vi "Depth and Stainless Correction Pop Up.vi"(2 "New Number\n of Stainless\n(Count)":i32, 3 "Input \nCorrected \nDepth (Feet)":sgl format="%.2f") -> (0 "Feet of\nStainless to be\nUsed (Count)":i32, 1 "Depth to \nbe Used \n(Feet)":sgl format="%.2f")   [LabVIEW 2016]
doc: "This vi allows the clinician to input the starting flexion. It used in order to derive a flexion correction."
panel:
  out "Original \nUncorrected \nDepth (Feet)":sgl format="%.2f"
  out "Original Feet\n of Stainless\n(Count)":i32
  in  "stop":bool
  in  "Increment Stainless":bool
  in  "Stainless OK As Is":bool
  in  "Correct Stainless":bool
  in  "Depth OK As Is":bool
  in  "Correct Depth":bool
  # "Please Choose \nto Correct Depth\nor to Leave As Is"
  # "Please Choose \nto Correct, Increment, or to \nLeave Feet of Stainless as is"
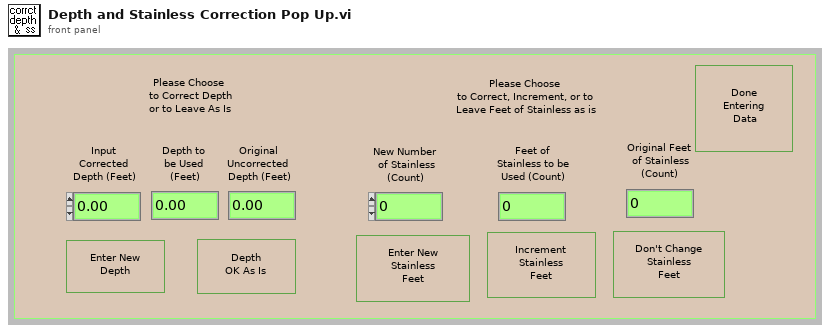
[diagram p1: front panel]
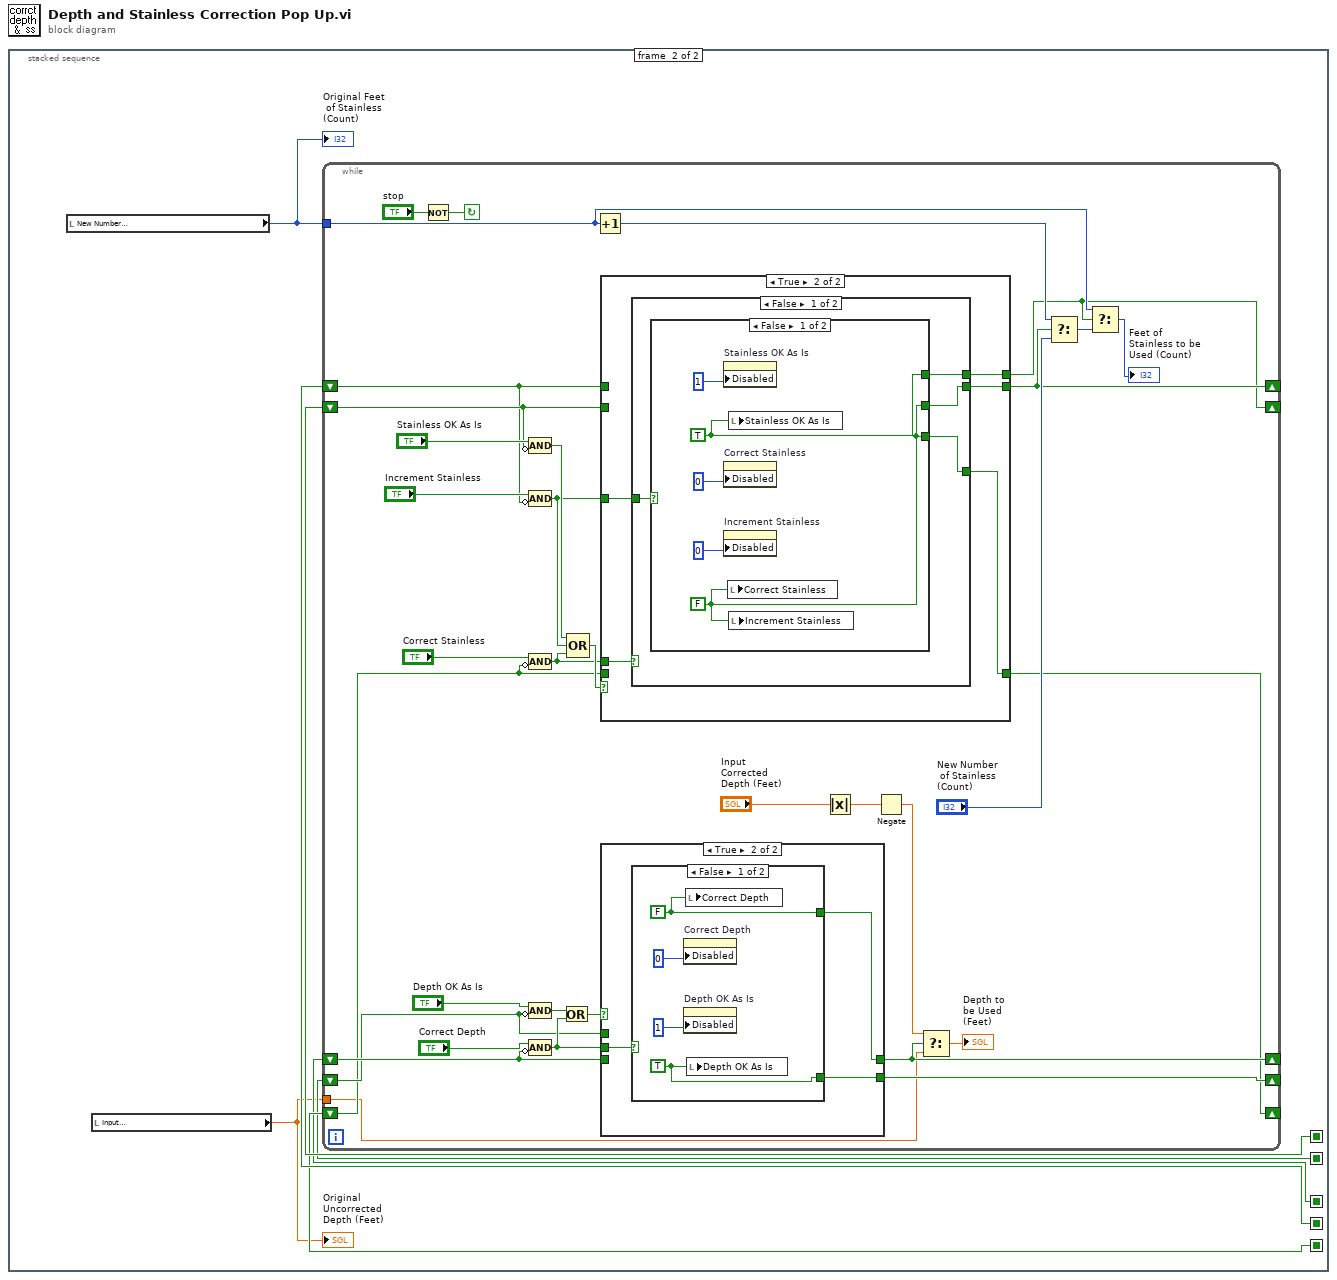
[diagram p0: block diagram]
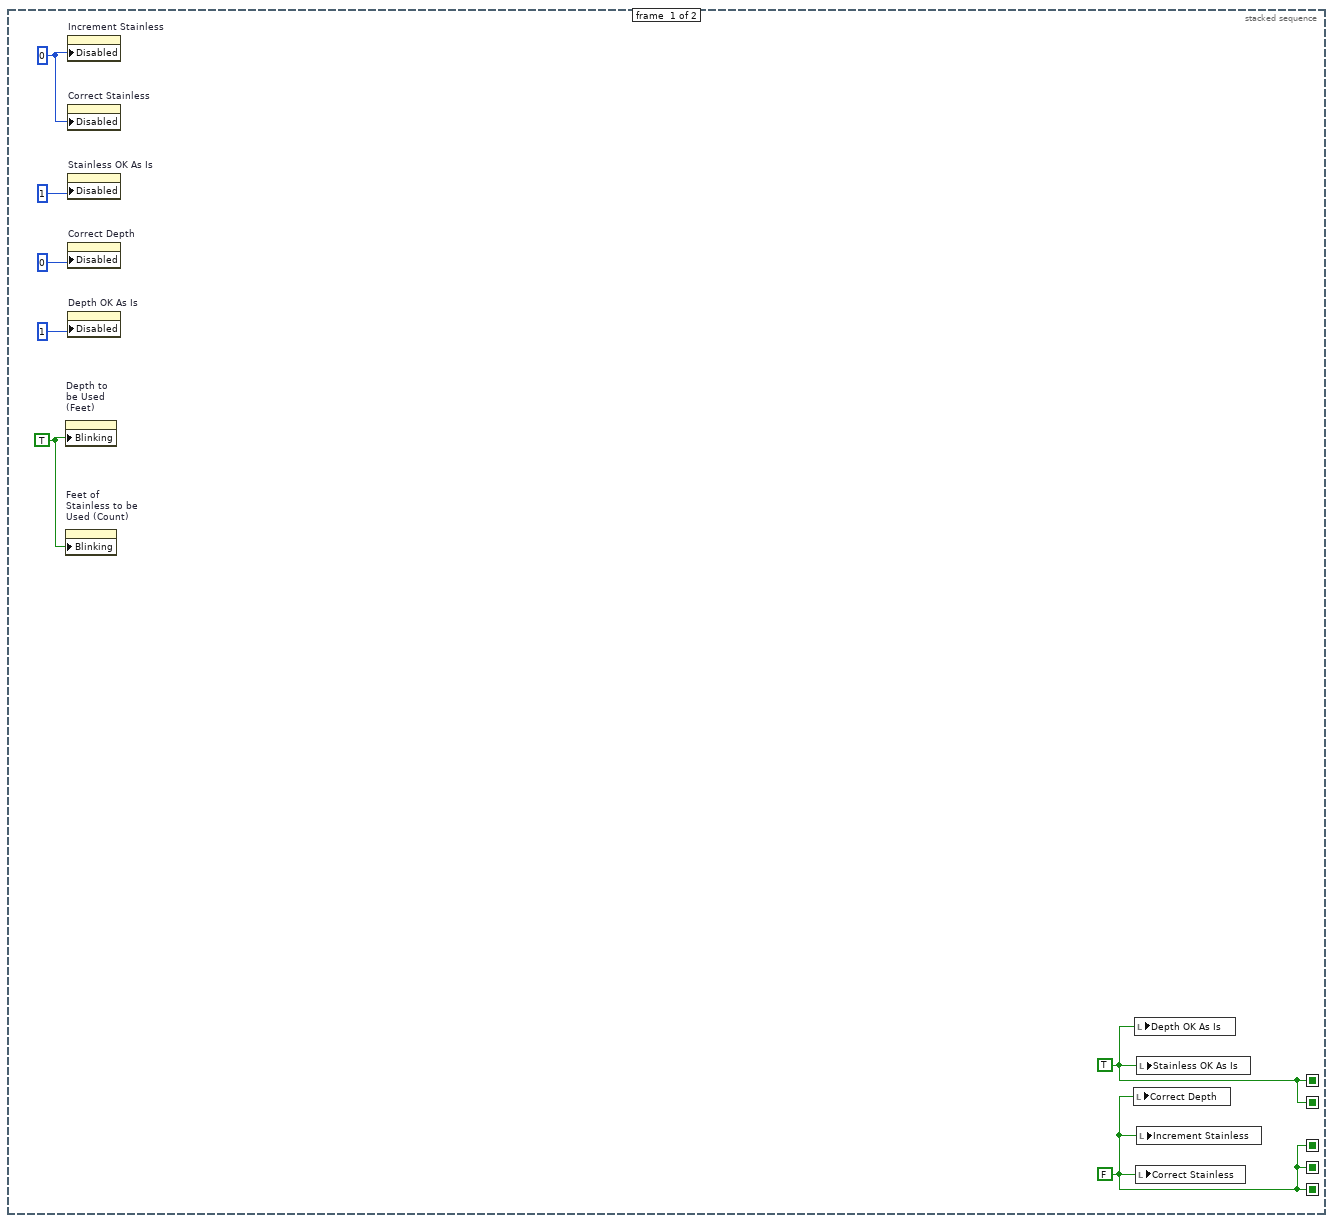
[diagram p2: hidden frame]
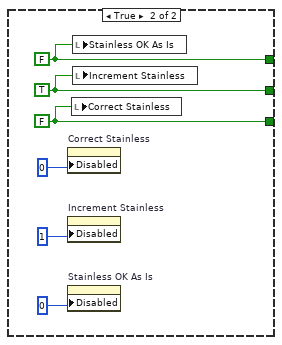
[diagram p4: hidden frame]
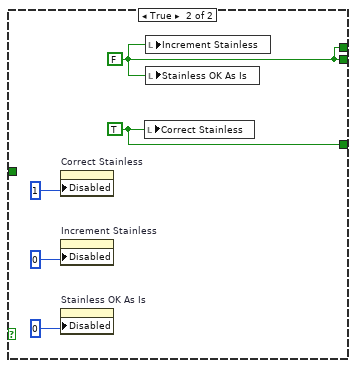
[diagram p5: hidden frame]
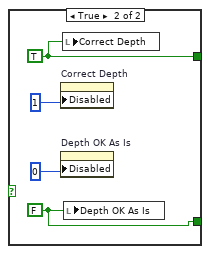
[diagram p7: hidden frame]
diagram:
  n1 = stacked-sequence {
    seq-local: [w6 _] -> [_ w12]
    seq-local: [w6 _] -> [_ w13]
    seq-local: [w7 _] -> [_ w14]
    seq-local: [w6 _] -> [_ w10]
    seq-local: [w7 _] -> [_ w11]
    frame #0 {
      w1 = TRUE
      w2 = 0
      w7 = TRUE
      w6 = FALSE
      n2 = property on="Depth to \nbe Used \n(Feet)" class="DigNum (strict)"("Blinking"=w1) -> ()  [unwired: 2 in, 2 out]
      n3 = property on="Feet of\nStainless to be\nUsed (Count)" class="DigNum (strict)"("Blinking"=w1) -> ()  [unwired: 2 in, 2 out]
      n4 = property on="Increment Stainless" class="Bool (strict)"("Disabled"=w2) -> ()  [unwired: 2 in, 2 out]
      n5 = property on="Correct Stainless" class="Bool (strict)"("Disabled"=w2) -> ()  [unwired: 2 in, 2 out]
      n6 = property on="Stainless OK As Is" class="Bool (strict)"("Disabled"=1) -> ()  [unwired: 2 in, 2 out]
      n7 = property on="Correct Depth" class="Bool (strict)"("Disabled"=0) -> ()  [unwired: 2 in, 2 out]
      n8 = property on="Depth OK As Is" class="Bool (strict)"("Disabled"=1) -> ()  [unwired: 2 in, 2 out]
      n9 = local write "Correct Depth"(w6) -> ()
      n10 = local write "Depth OK As Is"(w7) -> ()
      n11 = local write "Correct Stainless"(w6) -> ()
      n12 = local write "Stainless OK As Is"(w7) -> ()
      n13 = local write "Increment Stainless"(w6) -> ()
    }
    frame #1 {
      n14 = local read "New Number\n of Stainless\n(Count)"() -> (w9:i32)
      "Original Feet\n of Stainless\n(Count)" <- w9
      n15 = local read "Input \nCorrected \nDepth (Feet)"() -> (w8:sgl)
      "Original \nUncorrected \nDepth (Feet)" <- w8
      n16 = while {
        tunnel: w8 -> [w19]
        tunnel: w9 -> [w20]
        shift-left: w10 -> [w25]
        shift-right: [w36] -> _
        shift-left: w11 -> [w24]
        shift-right: [w37] -> _
        shift-left: w12 -> [w22]
        shift-right: [w29] -> _
        shift-left: w13 -> [w21]
        shift-right: [w30] -> _
        shift-left: w14 -> [w23]
        shift-right: [w18] -> _
        stop <- w26 continue-if-true
        n17 = Not(x="stop") -> (.not. x?=w26:bool)
        n18 = Compound Arithmetic op=AND("Stainless OK As Is", invert w23) -> (w32:bool)
        n19 = Compound Arithmetic op=AND("Increment Stainless", invert w21) -> (w27:bool)
        n20 = Compound Arithmetic op=AND("Correct Stainless", invert w22) -> (w28:bool)
        n21 = Compound Arithmetic op=AND("Depth OK As Is", invert w24) -> (w41:bool)
        n22 = Compound Arithmetic op=AND("Correct Depth", invert w25) -> (w39:bool)
        n23 = Or(x=w41, y=w39) -> (x .or. y?=w40:bool)
        n24 = Compound Arithmetic op=OR(w32, w27, w28) -> (w31:bool)
        n25 = Increment(x=w20) -> (x+1=w47:i32)
        n26 = case shown="True" w31 {
          tunnel: [w51 w54] -> w18
          tunnel: [w50 w53] -> w30
          tunnel: [w49 w55] -> w29
          tunnel: w28 -> [_ w56]
          tunnel: w27 -> [_ w52]
          tunnel: w23 -> [w51 _]
          tunnel: w22 -> [w49 _]
          tunnel: w21 -> [w50 _]
          frame False {
          }
          frame True {
            n27 = case shown="False" w56 {
              tunnel: [w57 w76] -> w55
              tunnel: [w59 w75] -> w54
              tunnel: [w58 w75] -> w53
              tunnel: w52 -> [w60 _]
              frame False {
                n28 = case shown="False" w60 {
                  tunnel: [w64 w69] -> w59
                  tunnel: [w65 w70] -> w58
                  tunnel: [w65 w71] -> w57
                  frame False {
                    w64 = TRUE
                    w65 = FALSE
                    n29 = property on="Stainless OK As Is" class="Bool (strict)"("Disabled"=1) -> ()  [unwired: 2 in, 2 out]
                    n30 = property on="Correct Stainless" class="Bool (strict)"("Disabled"=0) -> ()  [unwired: 2 in, 2 out]
                    n31 = property on="Increment Stainless" class="Bool (strict)"("Disabled"=0) -> ()  [unwired: 2 in, 2 out]
                    n32 = local write "Correct Stainless"(w65) -> ()
                    n33 = local write "Stainless OK As Is"(w64) -> ()
                    n34 = local write "Increment Stainless"(w65) -> ()
                  }
                  frame True {
                    w69 = FALSE
                    w70 = TRUE
                    w71 = FALSE
                    n35 = property on="Correct Stainless" class="Bool (strict)"("Disabled"=0) -> ()  [unwired: 2 in, 2 out]
                    n36 = property on="Increment Stainless" class="Bool (strict)"("Disabled"=1) -> ()  [unwired: 2 in, 2 out]
                    n37 = property on="Stainless OK As Is" class="Bool (strict)"("Disabled"=0) -> ()  [unwired: 2 in, 2 out]
                    n38 = local write "Correct Stainless"(w71) -> ()
                    n39 = local write "Stainless OK As Is"(w69) -> ()
                    n40 = local write "Increment Stainless"(w70) -> ()
                  }
                }
              }
              frame True {
                w75 = FALSE
                w76 = TRUE
                n41 = property on="Correct Stainless" class="Bool (strict)"("Disabled"=1) -> ()  [unwired: 2 in, 2 out]
                n42 = property on="Increment Stainless" class="Bool (strict)"("Disabled"=0) -> ()  [unwired: 2 in, 2 out]
                n43 = property on="Stainless OK As Is" class="Bool (strict)"("Disabled"=0) -> ()  [unwired: 2 in, 2 out]
                n44 = local write "Correct Stainless"(w76) -> ()
                n45 = local write "Increment Stainless"(w75) -> ()
                n46 = local write "Stainless OK As Is"(w75) -> ()
              }
            }
          }
        }
        n47 = case shown="True" w40 {
          tunnel: w39 -> [_ w81]
          tunnel: [w78 w79] -> w37
          tunnel: [w77 w80] -> w36
          tunnel: w25 -> [w77 _]
          tunnel: w24 -> [w78 _]
          frame False {
          }
          frame True {
            n48 = case shown="False" w81 {
              tunnel: [w85 w89] -> w80
              tunnel: [w84 w88] -> w79
              frame False {
                w85 = FALSE
                w84 = TRUE
                n49 = property on="Correct Depth" class="Bool (strict)"("Disabled"=0) -> ()  [unwired: 2 in, 2 out]
                n50 = property on="Depth OK As Is" class="Bool (strict)"("Disabled"=1) -> ()  [unwired: 2 in, 2 out]
                n51 = local write "Correct Depth"(w85) -> ()
                n52 = local write "Depth OK As Is"(w84) -> ()
              }
              frame True {
                w88 = FALSE
                w89 = TRUE
                n53 = property on="Correct Depth" class="Bool (strict)"("Disabled"=1) -> ()  [unwired: 2 in, 2 out]
                n54 = property on="Depth OK As Is" class="Bool (strict)"("Disabled"=0) -> ()  [unwired: 2 in, 2 out]
                n55 = local write "Correct Depth"(w89) -> ()
                n56 = local write "Depth OK As Is"(w88) -> ()
              }
            }
          }
        }
        n57 = Absolute Value(x="Input \nCorrected \nDepth (Feet)") -> (abs(x)=w16:sgl)
        n58 = Negate(x=w16) -> (-x=w15:sgl)
        n59 = Select(t=w15, s=w36, f=w19) -> (s? t:f=→"Depth to \nbe Used \n(Feet)":sgl)
        n60 = Select(t=w47, s=w30, f="New Number\n of Stainless\n(Count)") -> (s? t:f=w46:i32)
        n61 = Select(t=w20, s=w18, f=w46) -> (s? t:f=→"Feet of\nStainless to be\nUsed (Count)":i32)
      }
    }
  }
